vi "QControl Creator Core.vi"(8 "error in (no error)":errorcluster, 11 "New QControl Info":refnum<data-value>) -> (0 "error out":errorcluster)   [LabVIEW 2015, in "QControl Creation.lvclass"]
doc: "<b> </b> <b> </b>\n©2016 Q Software Innovations, LLC (QSI)\nwritten by Quentin Alldredge\nproduced in LabVIEW 2015\n\nsupport@qsoftwareinnovations.com\nwww.qsoftwareinnovations.com\n\nAll rights reserved.\n\nRedistribution and use in source and binary forms, with or without modification, are permitted provided that the following conditions are met:\n\n * Redistributions of source code must retain the above copyright notice, this list of conditions and the following disclaimer.\n * Redistributions in binary form must reproduce the above copyright notice, this list of conditions and the following disclaimer in the documentation and/or other materials provided with the distribution.\n * Neither the name of Q Software Innovations, LLC. nor the names of its contributors may be used to endorse or promote products derived from this software without specific prior written permission.\n\nTHIS SOFTWARE IS PROVIDED BY THE COPYRIGHT HOLDERS AND CONTRIBUTORS \"AS IS\" AND ANY EXPRESS OR IMPLIED WARRANTIES, INCLUDING, BUT NOT LIMITED TO, THE IMPLIED WARRANTIES OF MERCHANTABILITY AND FITNESS FOR A PARTICULAR PURPOSE ARE DISCLAIMED. IN NO EVENT SHALL THE COPYRIGHT OWNER OR CONTRIBUTORS BE LIABLE FOR ANY DIRECT, INDIRECT, INCIDENTAL, SPECIAL, EXEMPLARY, OR CONSEQUENTIAL DAMAGES (INCLUDING, BUT NOT LIMITED TO, PROCUREMENT OF SUBSTITUTE GOODS OR SERVICES; LOSS OF USE, DATA, OR PROFITS; OR BUSINESS INTERRUPTION) HOWEVER CAUSED AND ON ANY THEORY OF LIABILITY, WHETHER IN CONTRACT, STRICT LIABILITY, OR TORT (INCLUDING NEGLIGENCE OR OTHERWISE) ARISING IN ANY WAY OUT OF THE USE OF THIS SOFTWARE, EVEN IF ADVISED OF THE POSSIBILITY OF SUCH DAMAGE."
uses:
  QControl Creation.lvclass
  New QControl Info/New QControl Info.lvclass
  QControl Creation.lvclass/QControl Creation.ctl
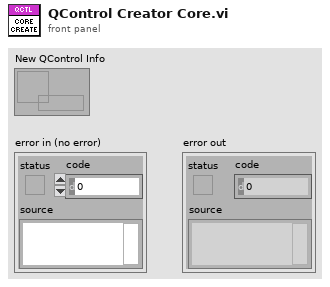
[diagram p1: front panel]
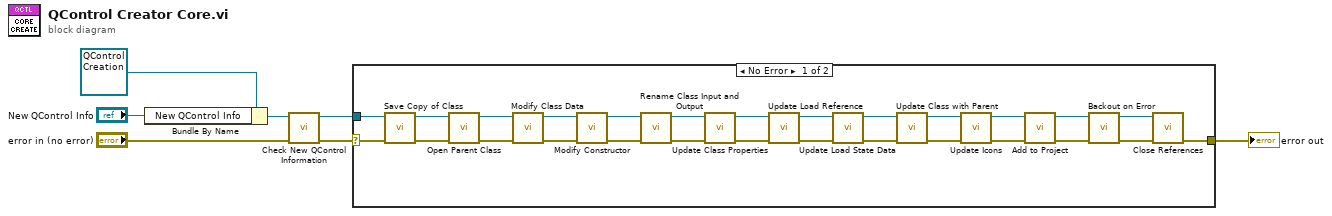
[diagram p0: block diagram]
diagram:
  n1 = Bundle By Name(cluster=refnum<class "QControl Creation.lvclass"> refnum ("QControl Creation in"), "New QControl Info"="New QControl Info") -> (w1:refnum<class "QControl Creation.lvclass">)
  n2 = call "Check New QControl Information.vi"("error in (no error)"="error in (no error)", "QControl Creation in"=w1) -> ("error out"=w4:errorcluster, "QControl Creation (dup)"=w6:refnum<class "QControl Creation.lvclass">)  [unwired: 8 in]
  n3 = case shown="No Error" w4 {
    selector: w4 -> [w34 w35]
    tunnel: [w12 w35] -> w7
    tunnel: w6 -> [w28 _]
    frame No Error {
      n4 = call "Save Copy of Class.vi"("error in (no error)"=w34, "QControl Creation in"=w28) -> ("error out"=w14:errorcluster, "QControl Creation out"=w16:refnum<class "QControl Creation.lvclass">)  [unwired: 8 in]
      n5 = call "Open Parent Class.vi"("error in (no error)"=w14, "QControl Creation in"=w16) -> ("error out"=w13:errorcluster, "QControl Creation out"=w15:refnum<class "QControl Creation.lvclass">)  [unwired: 8 in]
      n6 = call "Modify Class Data.vi"("error in (no error)"=w13, "QControl Creation in"=w15) -> ("error out"=w31:errorcluster, "QControl Creation (dup)"=w17:refnum<class "QControl Creation.lvclass">)  [unwired: 8 in]
      n7 = call "Modify Constructor.vi"("error in (no error)"=w31, "QControl Creation in"=w17) -> ("error out"=w30:errorcluster, "QControl Creation out"=w18:refnum<class "QControl Creation.lvclass">)  [unwired: 8 in]
      n8 = call "Rename Class Input and Output.vi"("error in (no error)"=w30, "QControl Creation in"=w18) -> ("error out"=w29:errorcluster, "QControl Creation (dup)"=w19:refnum<class "QControl Creation.lvclass">)  [unwired: 8 in]
      n9 = call "Update Class Properties.vi"("error in (no error)"=w29, "QControl Creation in"=w19) -> ("error out"=w32:errorcluster, "QControl Creation (dup)"=w20:refnum<class "QControl Creation.lvclass">)  [unwired: 8 in]
      n10 = call "Update Load Reference.vi"("error in (no error)"=w32, "QControl Creation in"=w20) -> ("error out"=w27:errorcluster, "QControl Creation (dup)"=w21:refnum<class "QControl Creation.lvclass">)  [unwired: 8 in]
      n11 = call "Update Load State Data.vi"("error in (no error)"=w27, "QControl Creation in"=w21) -> ("error out"=w26:errorcluster, "QControl Creation (dup)"=w22:refnum<class "QControl Creation.lvclass">)  [unwired: 8 in]
      n12 = call "Update Class with Parent.vi"("error in (no error)"=w26, "QControl Creation in"=w22) -> ("error out"=w25:errorcluster, "QControl Creation (dup)"=w23:refnum<class "QControl Creation.lvclass">)  [unwired: 8 in]
      n13 = call "Update Icons.vi"("error in (no error)"=w25, "QControl Creation in"=w23) -> ("error out"=w33:errorcluster, "QControl Creation (dup)"=w24:refnum<class "QControl Creation.lvclass">)  [unwired: 8 in]
      n14 = call "Add to Project.vi"("error in (no error)"=w33, "QControl Creation in"=w24) -> ("error out"=w9:errorcluster, "QControl Creation (dup)"=w8:refnum<class "QControl Creation.lvclass">)  [unwired: 8 in]
      n15 = call "Backout on Error.vi"("error in (no error)"=w9, "QControl Creation in"=w8) -> ("error out"=w10:errorcluster, "QControl Creation out"=w11:refnum<class "QControl Creation.lvclass">)  [unwired: 8 in]
      n16 = call "Close References.vi"("error in (no error)"=w10, "QControl Creation in"=w11) -> ("error out"=w12:errorcluster)  [unwired: 9 in]
    }
    frame Error {
    }
  }
  "error out" <- w7
